vi "getparray_v3.vi"(0 "IntensityGraph in":refnum<vi>, 1 "Metric Choice":bool, 2 "Frames number":i32=1, 3 "update M":dbl[][](array[numeric]), 4 "Use Cursor":bool, 5 "boxsize":i32=15) -> (6 "Array":dbl[](array[numeric]), 7 "subarray":u16[][](graph), 8 "sub subarray":u16[][](graph))   [LabVIEW 2015]
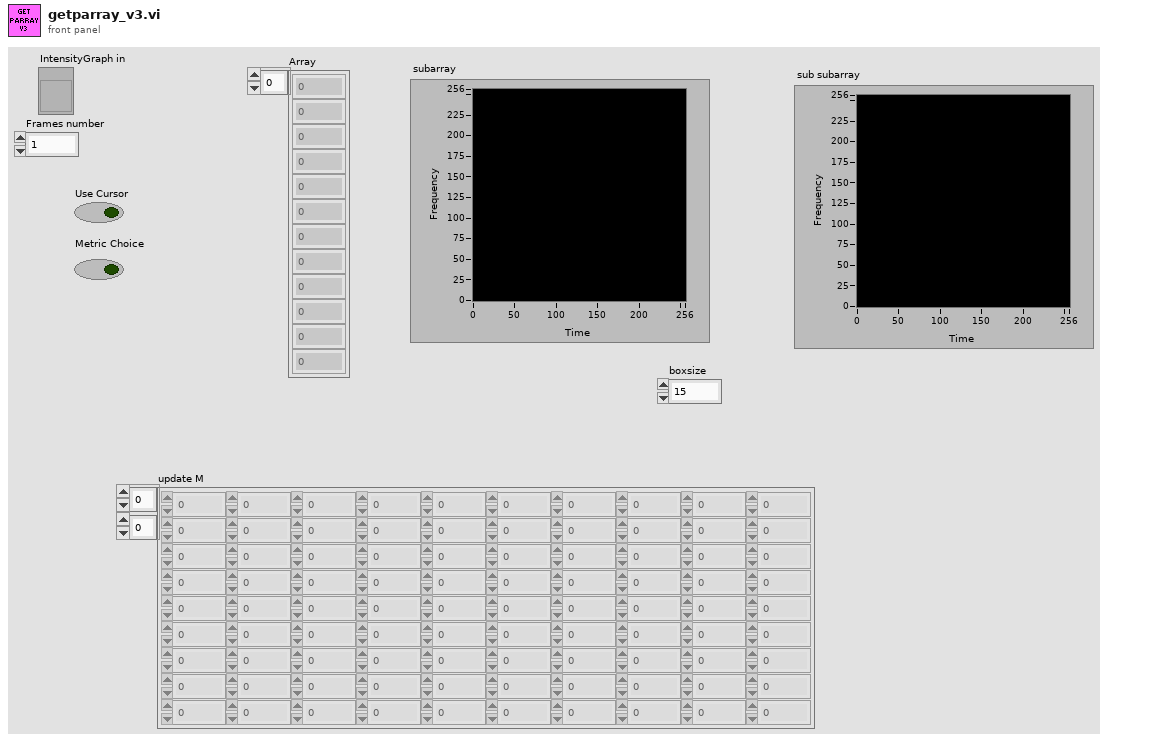
[diagram p1: front panel]
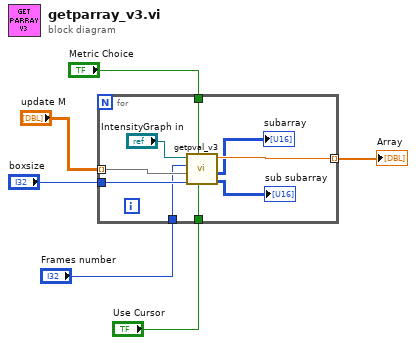
[diagram p0: block diagram]
diagram:
  n1 = for {
    tunnel: "update M" -> [w15] mode=indexing
    tunnel: [w14] -> w6 mode=indexing
    tunnel: "boxsize" -> [w13]
    tunnel: "Frames number" -> [w11]
    tunnel: "Metric Choice" -> [w10]
    tunnel: "Use Cursor" -> [w8]
    n2 = call "getpval_v3.vi"("Use Cursor"=w8, "Metric Choice"=w10, "boxsize"=w13, "amplitude"=w15, "Frames number"=w11, "IntensityGraph in"="IntensityGraph in") -> ("sub-subarray"=→"sub subarray":u16[][], "subarray"=→"subarray":u16[][], "pval"=w14:dbl)  [unwired: 1 out]
  }
  "Array" <- w6
